vi "FT10_Set Booleans to Disconnect.vi"(11 "Message Handling Cluster in":T1) -> (3 "Message Handling Cluster out":T1)   [LabVIEW 2024]
uses:
  Controls/Control_M4X Connection.ctl
  Controls/Control_PXI-7854R FPGA Reference.ctl
  Controls/Control_Message Handling Cluster.ctl
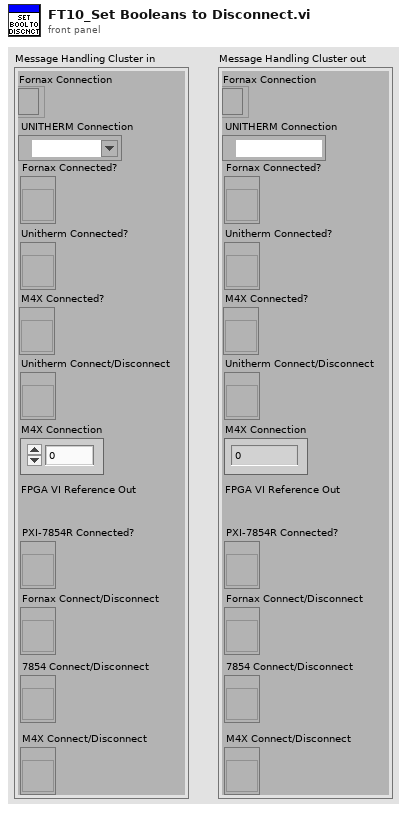
[diagram p1: front panel]
types:
  T1 = typedef "Control_Message Handling Cluster.ctl" = cluster{"Fornax Connected?":refnum<vi>, "Unitherm Connected?":refnum<vi>, "M4X Connected?":refnum<vi>, "Unitherm Connect/Disconnect":refnum<vi>, "Fornax Connection":refnum<k5>, "UNITHERM Connection":refnum<visa-resource-name>, "M4X Connection":T2, "PXI-7854R FPGA Reference":T3, "PXI-7854R Connected?":refnum<vi>, "Fornax Connect/Disconnect":refnum<vi>, "7854 Connect/Disconnect":refnum<vi>, "M4X Connect/Disconnect":refnum<vi>}
  T2 = typedef "Control_M4X Connection.ctl" = u32
  T3 = typedef "Control_PXI-7854R FPGA Reference.ctl" = refnum<k20>
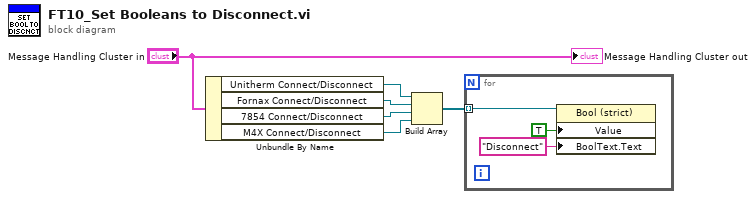
[diagram p0: block diagram]
diagram:
  n1 = Unbundle By Name("Message Handling Cluster in") -> ("Unitherm Connect/Disconnect"=w5:refnum<vi>, "Fornax Connect/Disconnect"=w4:refnum<vi>, "7854 Connect/Disconnect"=w3:refnum<vi>, "M4X Connect/Disconnect"=w2:refnum<vi>)
  n2 = Build Array(w5, w4, w3, w2) -> (w1:refnum<vi>[])
  n3 = for {
    tunnel: w1 -> [w7] mode=indexing
    n4 = property class="Bool (strict)"(reference=w7, "Value"=TRUE, "BoolText.Text"="Disconnect" ("Boolean Text.Text")) -> ()  [unwired: 1 in, 2 out]
  }
  "Message Handling Cluster out" <- "Message Handling Cluster in"
